vi "高级演示程序.vi"() -> ()   [LabVIEW 2012]
panel:
  out "存储中转":bool=TRUE
  in  "采样频率":i32=1000000
  in  "退出回放":bool
  out "zhongji":bool
  in  "退出系统":bool
  in  "触发时间":i32
  out "size":i32
  out "datafile":path[](array[path])
  in  "选项卡控件":enum32{"数据采集 ", "数字量采集", "数据回放"}(tab)
  out "实时波形显示":dbl[][](graph)
  out "当前状态":string
  in  "触发状态":bool
  in  "开始AD":bool
  in  "停止AD":bool
  in  "触发时间 2":i32 caption="mS"
  in  "定时":bool
  in  "触发按钮":bool
  in  "功能选项卡":enum32{"采集参数配置", "存储图形参数"}(tab)
  in  "M段":i32
  in  "N段":i32=40960
  in  "量程":T1(array[ring])
  in  "增益":enum16{"1倍", "2倍", "4倍", "8倍"}[](array[ring])
  in  "Y轴标尺调整":i8(knob) scale=0.0..10.0
  in  "文件名":string
  in  "存储":bool
  in  "触发方向":enum16{"下降沿触发", "上升沿触发", "上下边沿均触发"}(ring)
  in  "触发模式":enum16{"中间触发", "后触发", "预触发", "硬件延时触发"}(ring)
  in  "触发电平":i32
  in  "触发源":enum16{"软件触发", "DTR触发", "ATR触发", "Trig触发"}(ring)
  in  "时钟输出到总线":enum16{"不允许", "允许"}(ring)
  in  "时钟源":enum16{"内时钟", "外时钟"}(ring)
  in  "时钟输入输出源":T2(ring)
  in  "DO4":bool
  in  "DO5":bool
  in  "DO7":bool
  in  "DO6":bool
  in  "DO3":bool
  in  "DO2":bool
  in  "DO1":bool
  in  "DO0":bool
  out "DI7":bool
  out "DI6":bool
  out "DI5":bool
  out "DI4":bool
  out "DI3":bool
  out "DI2":bool
  out "DI1":bool
  out "DI0":bool
  in  "显示点数":u32(knob)=1000 min=1 max=10000 step=1000 scale=1.0..10000.0
  in  "刷新速度":u32(knob)=100 min=100 max=1000 step=100 scale=100.0..1000.0
  in  "开始":bool
  out "Waveform Graph 3":dbl[](graph)
  in  "导入":bool
  in  "循环速度（MS）":u32=300
  in  "量程-1":T3(ring)
  # "时钟源"
  # "触发方式"
  # "通道设置"
  # "数字量输出"
  # "数字量采集"
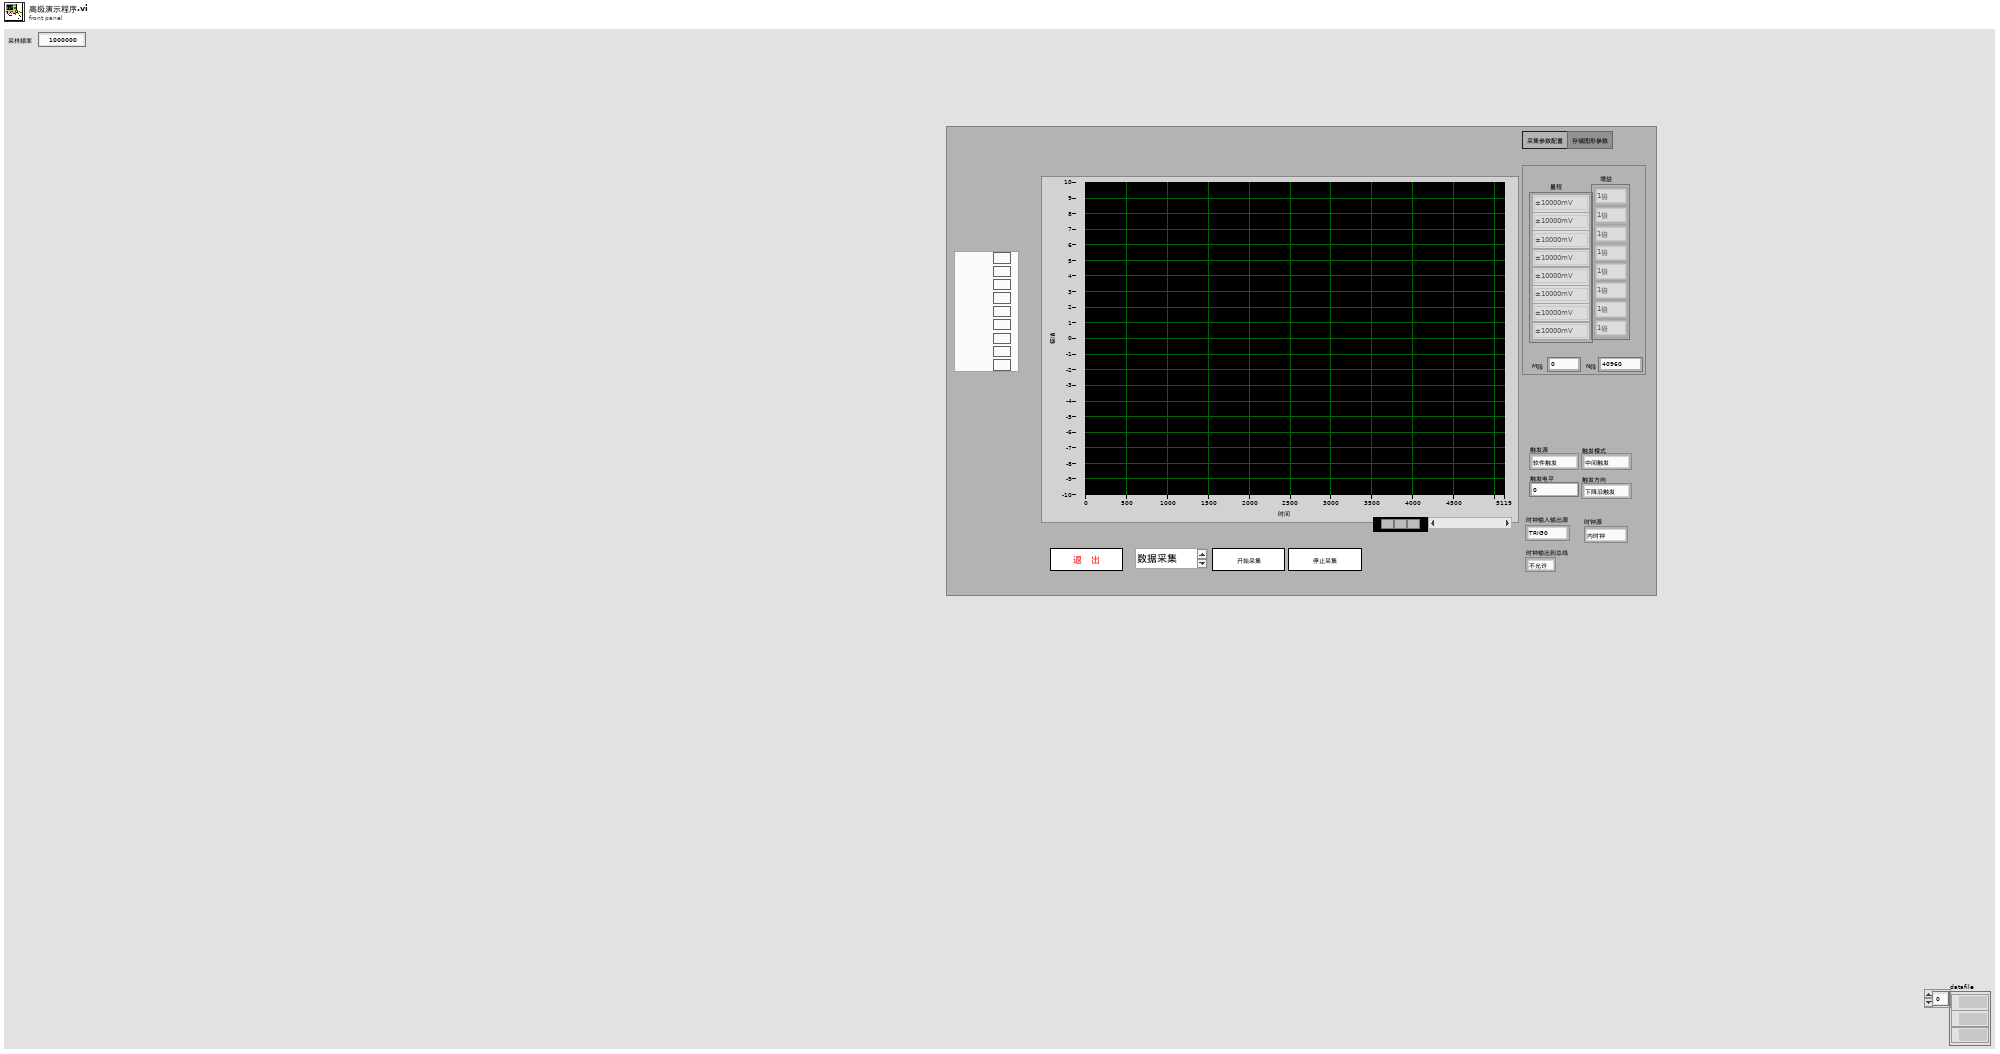
[diagram p1: front panel]
types:
  T1 = enum16{"±10000mV", "±5000mV", "±2500mV", "0-10000mV", "0-5000mV"}[]
  T2 = enum16{"TRIG0", "TRIG1", "TRIG2", "TRIG3", "TRIG4", "TRIG5", "TRIG6", "TRIG7"}
  T3 = enum16{"±10000mV", "±5000mV", "±2500mV", "0-10000mV", "0-5000mV"}
  T4 = enum8{"Enabled", "Disabled", "Disabled and Grayed Out"}
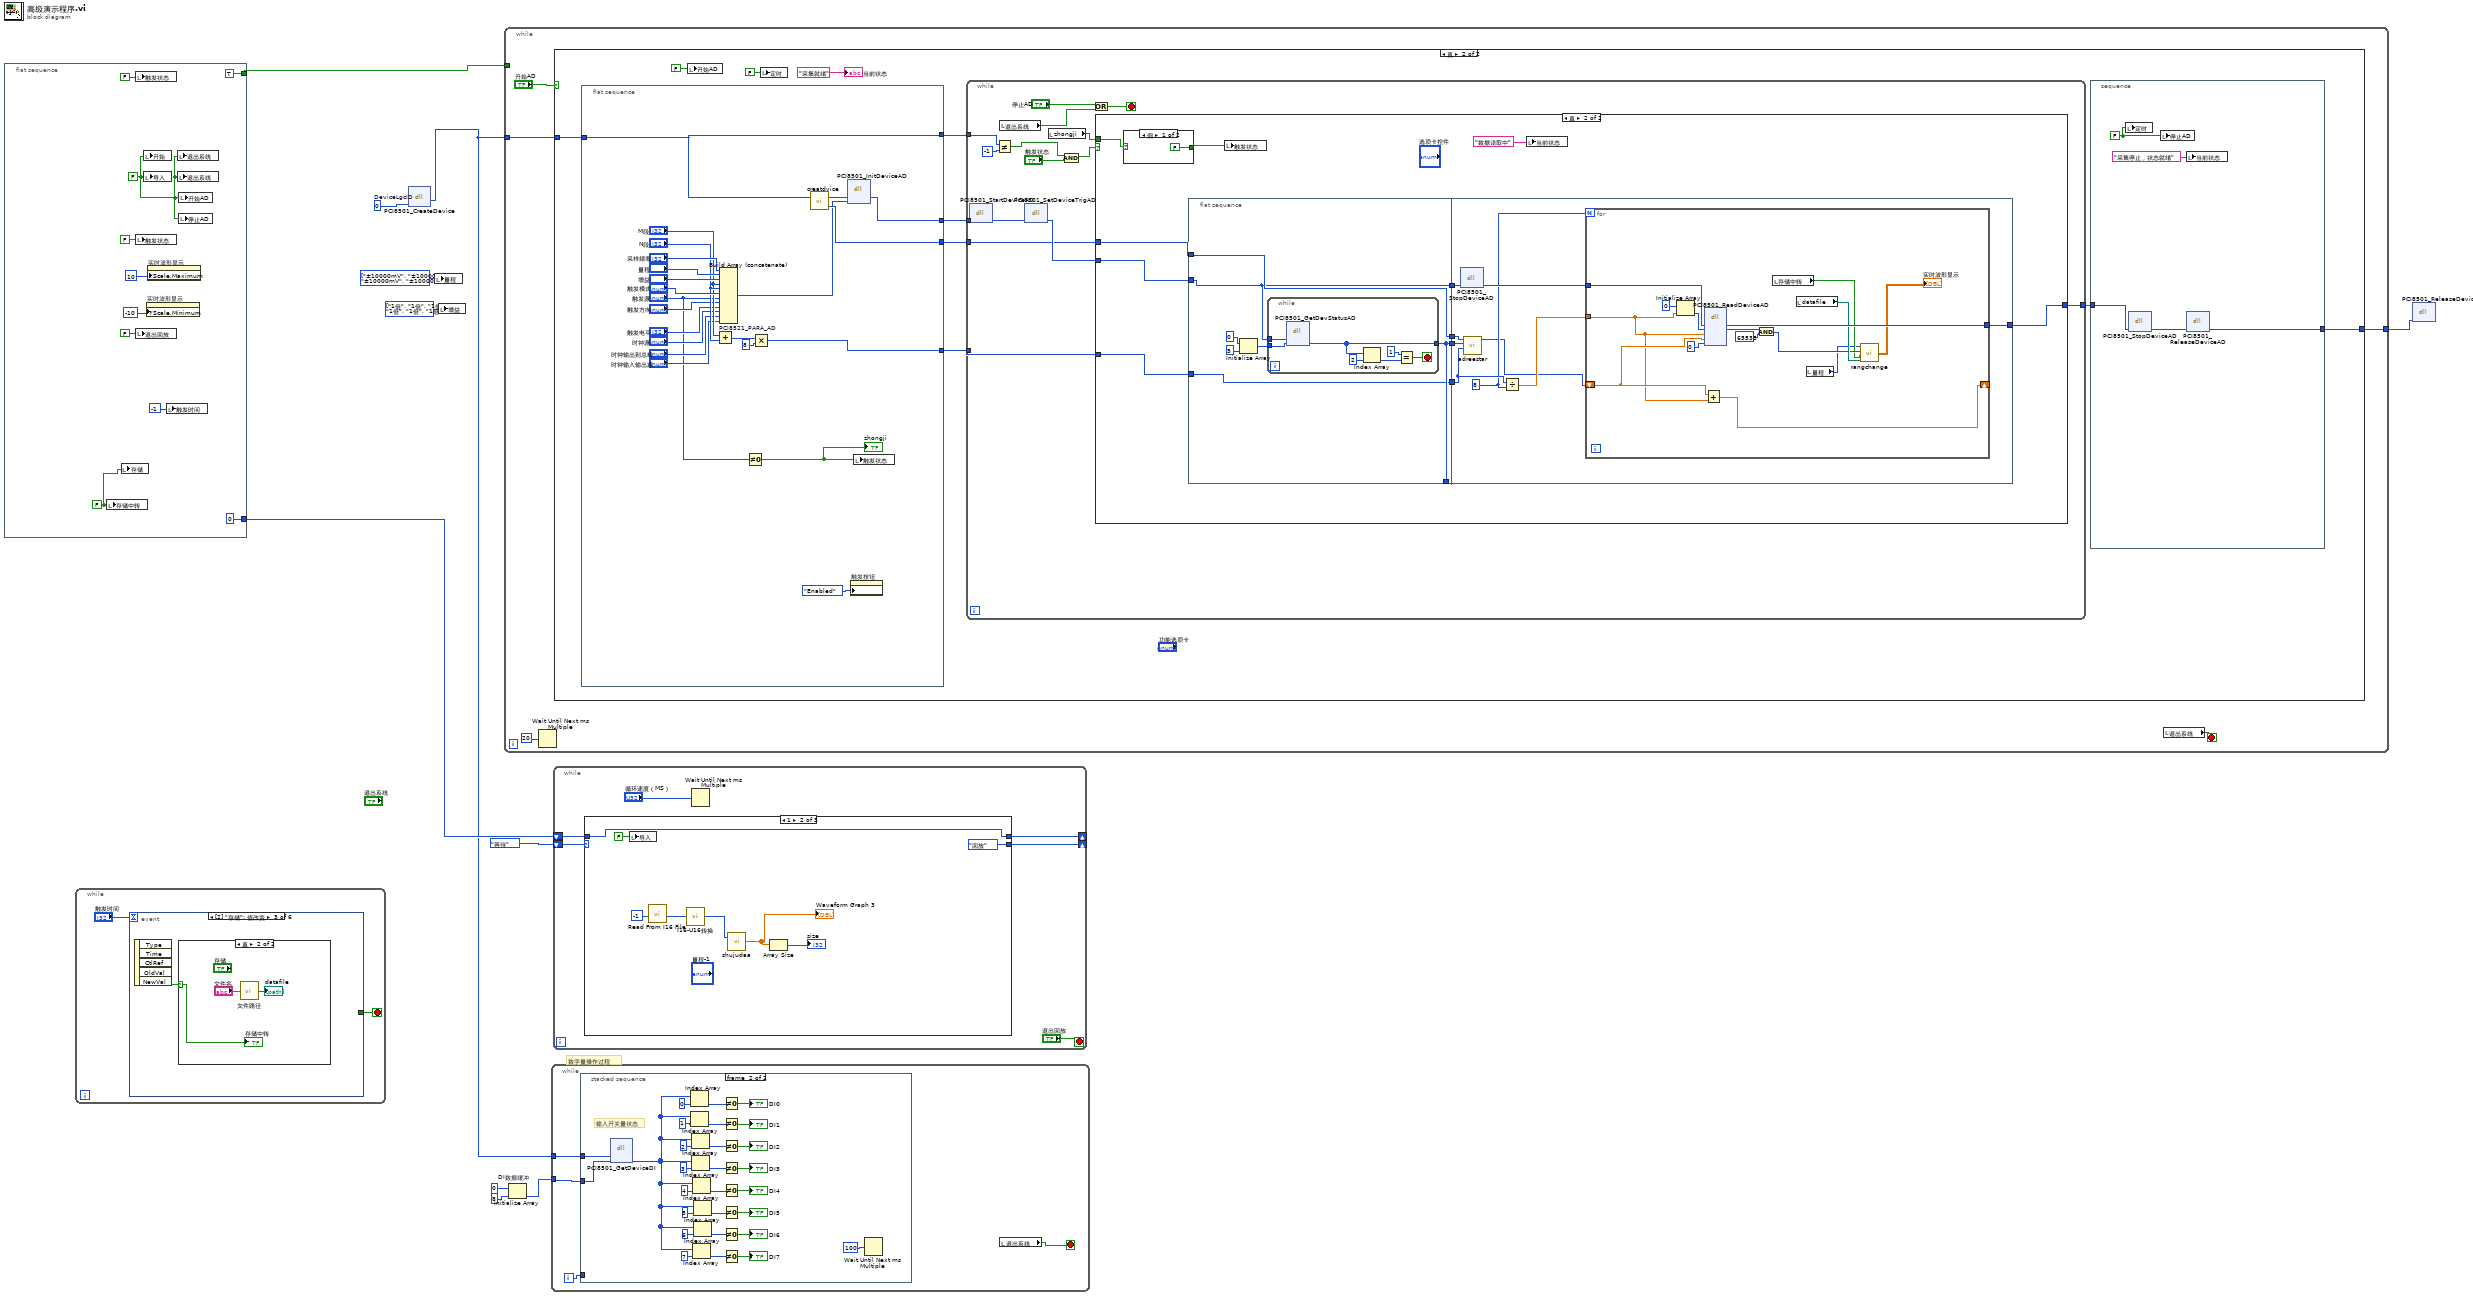
[diagram p0: block diagram]
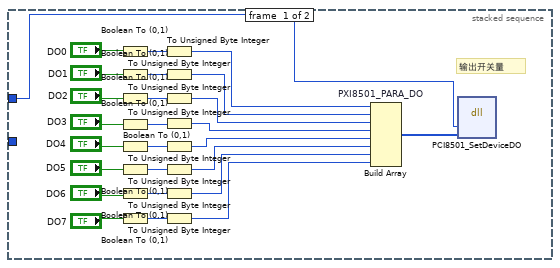
[diagram p2: hidden frame]
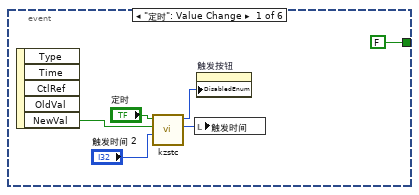
[diagram p3: hidden frame]
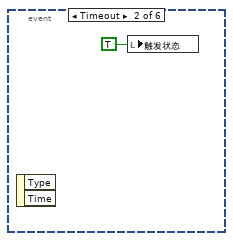
[diagram p4: hidden frame]
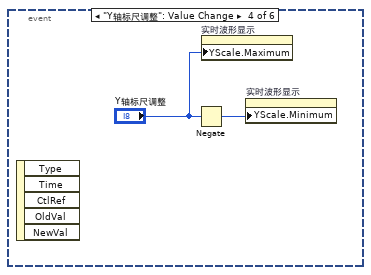
[diagram p6: hidden frame]
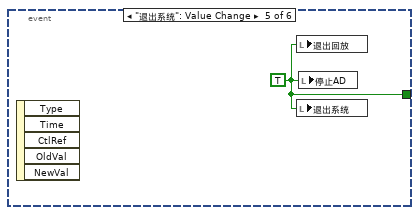
[diagram p7: hidden frame]
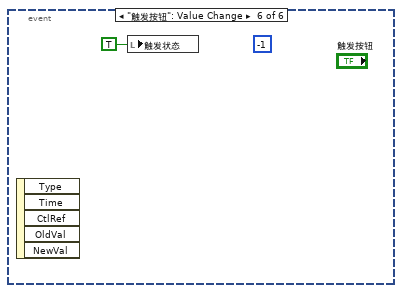
[diagram p8: hidden frame]
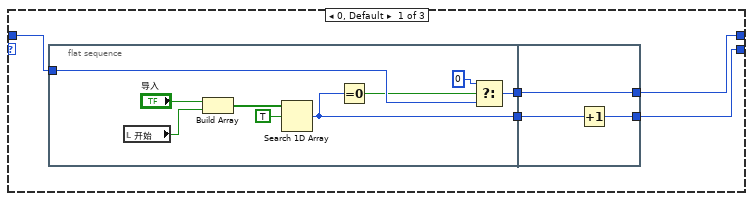
[diagram p9: hidden frame]
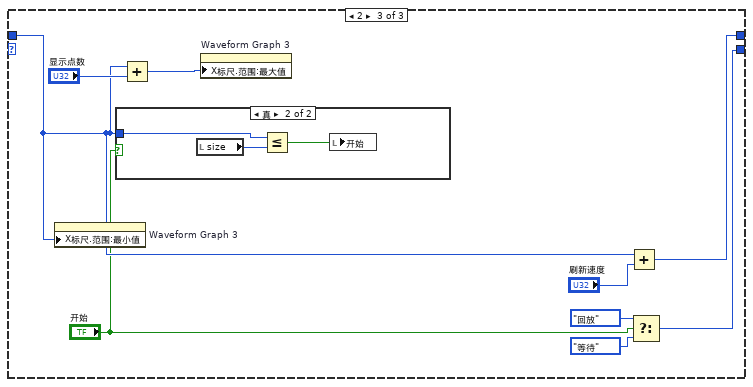
[diagram p10: hidden frame]
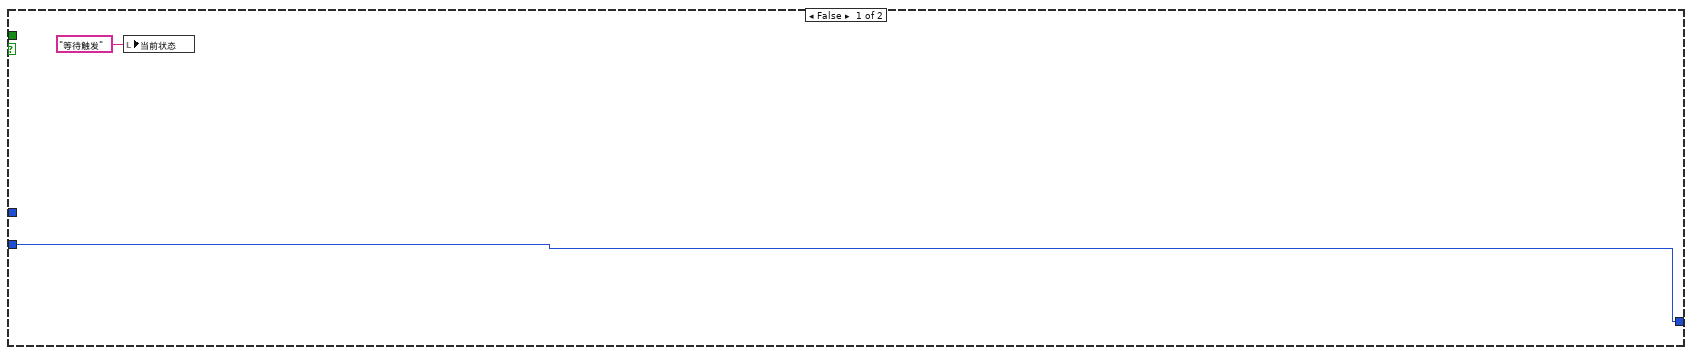
[diagram p13: hidden frame]
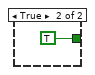
[diagram p14: hidden frame]
diagram:
  w1 = enum16{"1倍", "2倍", "4倍", "8倍"}[] [enum."1倍", enum."1倍", enum."1倍", enum."1倍", enum."1倍", enum."1倍", enum."1倍", enum."1倍"] items=["1倍", "2倍", "4倍", "8倍"] ("增益")
  w2 = T1 [enum."±10000mV", enum."±10000mV", enum."±10000mV", enum."±10000mV", enum."±10000mV", enum."±10000mV", enum."±10000mV", enum."±10000mV"] items=["±10000mV", "±5000mV", "±2500mV", "0-10000mV", "0-5000mV"] ("量程")
  w4 = 0  # DeviceLgcID
  # "数字量操作过程"
  n1 = flat-sequence {
    tunnel: [TRUE] -> w10
    tunnel: [0] -> w6
    frame #0 {
      w12 = FALSE ("存储中转")
      w18 = FALSE ("开始AD")
      n2 = local write "存储中转"(w12) -> ()
      n3 = local write "存储"(w12) -> ()
      n4 = local write "触发状态"(FALSE ("tirg")) -> ()
      n5 = local write "触发状态"(FALSE ("触发状态")) -> ()
      n6 = local write "退出回放"(FALSE ("退出回放")) -> ()
      n7 = local write "开始"(w18) -> ()
      n8 = local write "导入"(w18) -> ()
      n9 = property on="实时波形显示" class="WFGraph (严格)"("YScale.Minimum"=i8 -10 ("Y标尺.范围:最小值")) -> ()  [unwired: 2 in, 2 out]
      n10 = property on="实时波形显示" class="WFGraph (严格)"("YScale.Maximum"=u8 10 ("Y标尺.范围:最大值")) -> ()  [unwired: 2 in, 2 out]
      n11 = local write "触发时间"(-1 ("触发时间 2")) -> ()
      n12 = local write "退出系统"(w18) -> ()
      n13 = local write "退出系统"(w18) -> ()
      n14 = local write "开始AD"(w18) -> ()
      n15 = local write "停止AD"(w18) -> ()
    }
  }
  n16 = while {
    stop <- w23 stop-if-true
    n17 = event shown="[2] \"存储\": 值改变" {
      selector: _ -> [_ _ _ _ _ _]
      dyn-events: _ -> [_ _ _ _ _ _]
      timeout: "触发时间" -> [_ _ _ _ _ _]
      tunnel: [FALSE _ _ _ w37 _] -> w23
      event "定时": Value Change {
        n18 = event-data() -> ("NewVal"=w27:bool)  [unwired: 1 in, 4 out]
        n19 = call "kzstc.vi"("触发时间输入"="触发时间 2", "NewVal"=w27, "定时"="定时") -> ("触发时间输出"=w28:i32, "禁用"=w26:T4)  [unwired: 7 in]
        n20 = local write "触发时间"(w28) -> ()
        n21 = property on="触发按钮" class="Bool"("DisabledEnum"=w26) -> ()  [unwired: 2 in, 2 out]
      }
      event Timeout {
        n22 = event-data() -> ()  [unwired: 1 in, 2 out]
        n23 = local write "触发状态"(TRUE ("tirg")) -> ()
      }
      event "存储": Value Change {
        n24 = event-data() -> ("NewVal"=w31:bool)  [unwired: 1 in, 4 out]
        n25 = case shown="真" w31 {
          selector: w31 -> [_ w32]
          frame False {
          }
          frame True {
            n26 = call "文件路径.vi"("文件名"="文件名") -> ("数组"=→"datafile":path[])
            "存储中转" <- w32
          }
        }
      }
      event "Y轴标尺调整": Value Change {
        n27 = event-data() -> ()  [unwired: 1 in, 5 out]
        n28 = Negate(x="Y轴标尺调整") -> (-x=w36:i8)
        n29 = property on="实时波形显示" class="WFGraph (严格)"("YScale.Maximum"="Y轴标尺调整") -> ()  [unwired: 2 in, 2 out]
        n30 = property on="实时波形显示" class="WFGraph (严格)"("YScale.Minimum"=w36) -> ()  [unwired: 2 in, 2 out]
      }
      event "退出系统": Value Change {
        w37 = TRUE
        n31 = event-data() -> ()  [unwired: 1 in, 5 out]
        n32 = local write "退出回放"(w37) -> ()
        n33 = local write "退出系统"(w37) -> ()
        n34 = local write "停止AD"(w37) -> ()
      }
      event "触发按钮": Value Change {
        (unwired) -1 ("触发时间")
        n35 = event-data() -> ()  [unwired: 1 in, 5 out]
        n36 = local write "触发状态"(TRUE ("tirg")) -> ()
      }
    }
  }
  n37 = dll-call lib="PCI8501_32" fn="PCI8501_CreateDevice" label="CreateDevice"("DeviceLgcID"=w4) -> ("返回类型"=w3:i32)  [unwired: 4 in, 2 out]
  n38 = local write "量程"(w2) -> ()
  n39 = local write "增益"(w1) -> ()
  n40 = while {
    tunnel: w10 -> [_]
    tunnel: [w40] -> w5
    tunnel: w3 -> [w39]
    stop <- w43 stop-if-true
    n41 = Wait Until Next ms Multiple(millisecond multiple=u32 20 ("毫秒倍数")) -> ()  [unwired: 1 out]
    n42 = case shown="真" "开始AD" {
      tunnel: [_ w46] -> w40
      tunnel: w39 -> [_ w45]
      frame False {
      }
      frame True {
        n43 = flat-sequence {
          tunnel: [w55] -> w53
          tunnel: [w72] -> w49
          tunnel: [w71] -> w48
          tunnel: w45 -> [w70]
          tunnel: [w70] -> w44
          frame #0 {
            n44 = Add(x="M段", y="N段") -> (x+y=w69:i32)
            n45 = Build Array (concatenate) "PCI8521_PARA_AD"("采样频率", "量程", "增益", "M段", "N段", "触发模式", "触发源", "触发方向", "触发电平", "时钟源", "时钟输出到总线", "时钟输入输出源") -> (w56:i32[])
            n46 = Not Equal To 0?(x="触发源") -> (x != 0?=w75:bool)
            "zhongji" <- w75
            n47 = Multiply(x=w69, y=8 ("element")) -> (x*y=w55:i32)
            n48 = call "creatdvice.vi"("数值"=w70) -> ("ddrlength"=w71:i32, "hDevice"=w73:i32)  [unwired: 1 in]
            n49 = dll-call lib="PCI8501_32" fn="PCI8501_InitDeviceAD" label="InitDeviceAD"("hDevice"=w73, "pADPara"=w56) -> ("hDevice"=w72:i32)  [unwired: 5 in, 2 out]
            n50 = property on="触发按钮" class="Bool"("DisabledEnum"=T4."Enabled" ("禁用")) -> ()  [unwired: 2 in, 2 out]
            n51 = local write "触发状态"(w75) -> ()
          }
        }
        n52 = local write "开始AD"(FALSE ("开始AD")) -> ()
        n53 = local write "定时"(FALSE ("定时")) -> ()
        n54 = while {
          tunnel: w53 -> [w78]
          tunnel: w49 -> [w81]
          tunnel: w48 -> [w79]
          tunnel: [w77] -> w47
          tunnel: w44 -> [w76]
          stop <- w87 stop-if-true
          n55 = dll-call lib="PCI8501_32" fn="PCI8501_StartDeviceAD" label="StartDeviceAD"("hDevice"=w81) -> ("hDevice"=w82:i32)  [unwired: 4 in, 2 out]
          n56 = Not Equal?(x=w76, y=-1) -> (x != y?=w86:bool)
          n57 = local read "退出系统"() -> (w88:bool)
          n58 = dll-call lib="PCI8501_32" fn="PCI8501_SetDeviceTrigAD" label="SetDeviceTrigAD"("hDevice"=w82) -> ("hDevice"=w80:i32)  [unwired: 4 in, 2 out]
          n59 = local read "zhongji"() -> (w83:bool)
          n60 = Compound Arithmetic op=AND(w86, "触发状态") -> (w85:bool)
          n61 = Or(x="停止AD", y=w88) -> (x .or. y?=w87:bool)
          n62 = case shown="真" w85 {
            tunnel: w83 -> [_ w102]
            tunnel: w80 -> [w91 w96]
            tunnel: w79 -> [_ w95]
            tunnel: w78 -> [_ w94]
            tunnel: [w91 w93] -> w77
            frame False {
              n63 = local write "当前状态"("等待触发" ("当前状态")) -> ()
            }
            frame True {
              n64 = case shown="假" w102 {
                tunnel: [FALSE ("触发状态") TRUE ("触发状态")] -> w103
                frame False {
                }
                frame True {
                }
              }
              n65 = flat-sequence {
                tunnel: [w104] -> w100
                tunnel: [w107] -> _
                tunnel: w94 -> [w106]
                tunnel: [w106] -> w99
                tunnel: w95 -> [w105]
                tunnel: [w105] -> w98
                tunnel: [w107] -> w97
                tunnel: w96 -> [w104]
                tunnel: w100 -> [w126]
                tunnel: [w124] -> w93
                tunnel: w99 -> [w121]
                tunnel: w98 -> [w122]
                tunnel: w97 -> [w123]
                frame #0 {
                  n66 = Initialize Array(0, 5) -> (w110:i32[])
                  n67 = while {
                    tunnel: w104 -> [w117]
                    tunnel: w110 -> [w116]
                    tunnel: [w111] -> w107
                    stop <- w112 stop-if-true
                    n68 = dll-call lib="PCI8501_32" fn="PCI8501_GetDevStatusAD" label="GetDevStatusAD"("hDevice"=w117, "ADStatus"=w116) -> ("ADStatus"=w111:i32[])  [unwired: 5 in, 2 out]
                    n69 = Index Array(array=w111, index=2) -> (element=w114:i32)
                    n70 = Equal?(x=1, y=w114) -> (x = y?=w112:bool)
                  }
                }
                frame #1 {
                  w120 = 8 ("y")
                  n71 = dll-call lib="PCI8501_32" fn="PCI8501_StopDeviceAD" label="StopDeviceAD"("hDevice"=w126) -> ("hDevice"=w125:i32)  [unwired: 4 in, 2 out]
                  n72 = call "adreestar.vi"("M+N*8"=w121, "ADStatus"=w123, "ddrlength"=w122) -> ("adree"=w118:i32)  [unwired: 8 in]
                  n73 = Divide(x=w121, y=w120) -> (x/y=w119:dbl)
                  n74 = for {
                    N: w120 -> [_]
                    tunnel: w125 -> [w137]
                    tunnel: [w135] -> w124
                    shift-right: [w132] -> _
                    shift-left: w118 -> [w134]
                    tunnel: w119 -> [w133]
                    n75 = Initialize Array(0 ("y"), w133) -> (w139:i32[])
                    n76 = dll-call lib="PCI8501_32" fn="PCI8501_ReadDeviceAD" label="ReadDeviceAD"("hDevice"=w137, "ADBuffer"=w139, "AD_DATA_LEN"=w133, "ulStartAddr"=w134, "nRetSizeWords"=0 ("y")) -> ("hDevice"=w135:i32, "ADBuffer"=w136:u16[])  [unwired: 7 in, 2 out]
                    n77 = Add(x=w134, y=w133) -> (x+y=w132:dbl)
                    n78 = And(x=w136, y=65535) -> (x .and. y?=w129:i32[])
                    n79 = local read "存储中转"() -> (w128:bool)
                    n80 = local read "datafile"() -> (w131:path[])
                    n81 = local read "量程"() -> (w127:T1)
                    n82 = call "rangchange.vi"("datafile"=w131, "savaen"=w128, "IN"=w129, "添加的数组 2"=w127) -> ("添加的数组"=→"实时波形显示":dbl[][])  [unwired: 2 in]
                  }
                }
              }
              n83 = local write "触发状态"(w103) -> ()
              n84 = local write "当前状态"("数据读取中" ("当前状态")) -> ()
            }
          }
        }
        n85 = stacked-sequence {
          tunnel: w47 -> [w145]
          tunnel: [w144] -> w46
          frame #0 {
            w148 = FALSE ("停止AD")
            n86 = local write "定时"(w148) -> ()
            n87 = dll-call lib="PCI8501_32" fn="PCI8501_StopDeviceAD" label="StopDeviceAD"("hDevice"=w145) -> ("hDevice"=w146:i32)  [unwired: 4 in, 2 out]
            n88 = local write "停止AD"(w148) -> ()
            n89 = local write "当前状态"("采集停止，状态就绪" ("当前状态")) -> ()
            n90 = dll-call lib="PCI8501_32" fn="PCI8501_ReleaseDeviceAD" label="ReleaseDeviceAD"("hDevice"=w146) -> ("hDevice"=w144:i32)  [unwired: 4 in, 2 out]
          }
        }
        "当前状态" <- "采集就绪" ("当前状态")
      }
    }
    n91 = local read "退出系统"() -> (w43:bool)
  }
  n92 = Initialize Array "DI数据缓冲"(u8 0 ("元素初值"), 8) -> (w7:u8[])
  n93 = while {
    tunnel: w7 -> [w152]
    tunnel: w3 -> [w149]
    i -> [w151]
    stop <- w150 stop-if-true
    n94 = stacked-sequence {
      tunnel: w152 -> [_ w182]
      tunnel: w151 -> [_ _]
      tunnel: w149 -> [w153 w179]
      frame #0 {
        # "输出开关量"
        n95 = Boolean To (0,1)(Boolean="DO0") -> (0, 1=w170:i16)
        n96 = Boolean To (0,1)(Boolean="DO1") -> (0, 1=w178:i16)
        n97 = Boolean To (0,1)(Boolean="DO2") -> (0, 1=w175:i16)
        n98 = Boolean To (0,1)(Boolean="DO3") -> (0, 1=w169:i16)
        n99 = Boolean To (0,1)(Boolean="DO4") -> (0, 1=w174:i16)
        n100 = Boolean To (0,1)(Boolean="DO5") -> (0, 1=w173:i16)
        n101 = Boolean To (0,1)(Boolean="DO6") -> (0, 1=w172:i16)
        n102 = Boolean To (0,1)(Boolean="DO7") -> (0, 1=w171:i16)
        n103 = To Unsigned Byte Integer(number=w170) -> (unsigned 8bit integer=w168:u8)
        n104 = To Unsigned Byte Integer(number=w178) -> (unsigned 8bit integer=w167:u8)
        n105 = To Unsigned Byte Integer(number=w175) -> (unsigned 8bit integer=w166:u8)
        n106 = To Unsigned Byte Integer(number=w169) -> (unsigned 8bit integer=w165:u8)
        n107 = To Unsigned Byte Integer(number=w174) -> (unsigned 8bit integer=w164:u8)
        n108 = To Unsigned Byte Integer(number=w173) -> (unsigned 8bit integer=w163:u8)
        n109 = To Unsigned Byte Integer(number=w172) -> (unsigned 8bit integer=w162:u8)
        n110 = To Unsigned Byte Integer(number=w171) -> (unsigned 8bit integer=w161:u8)
        n111 = Build Array "PXI8501_PARA_DO"(w168, w167, w166, w165, w164, w163, w162, w161) -> (w154:u8[])
        n112 = dll-call lib="PCI8501_32" fn="PCI8501_SetDeviceDO" label="SetDeviceDO"("hDevice"=w153, "bDOSts"=w154) -> ()  [unwired: 6 in, 2 out]
      }
      frame #1 {
        # "输入开关量状态"
        n113 = dll-call lib="PCI8501_32" fn="PCI8501_GetDeviceDI" label="GetDeviceDI"("hDevice"=w179, "bDISts"=w182) -> ("bDISts"=w181:u8[])  [unwired: 5 in, 2 out]
        n114 = Index Array(array=w181, index=0) -> (element=w197:u8)
        n115 = Index Array(array=w181, index=1) -> (element=w198:u8)
        n116 = Index Array(array=w181, index=2) -> (element=w196:u8)
        n117 = Index Array(array=w181, index=3) -> (element=w195:u8)
        n118 = Index Array(array=w181, index=4) -> (element=w194:u8)
        n119 = Index Array(array=w181, index=7) -> (element=w191:u8)
        n120 = Index Array(array=w181, index=5) -> (element=w193:u8)
        n121 = Index Array(array=w181, index=6) -> (element=w192:u8)
        n122 = Not Equal To 0?(x=w197) -> (x != 0?=→"DI0":bool)
        n123 = Not Equal To 0?(x=w198) -> (x != 0?=→"DI1":bool)
        n124 = Not Equal To 0?(x=w196) -> (x != 0?=→"DI2":bool)
        n125 = Not Equal To 0?(x=w195) -> (x != 0?=→"DI3":bool)
        n126 = Not Equal To 0?(x=w194) -> (x != 0?=→"DI4":bool)
        n127 = Not Equal To 0?(x=w193) -> (x != 0?=→"DI5":bool)
        n128 = Not Equal To 0?(x=w192) -> (x != 0?=→"DI6":bool)
        n129 = Not Equal To 0?(x=w191) -> (x != 0?=→"DI7":bool)
        n130 = Wait Until Next ms Multiple(millisecond multiple=u32 100) -> ()  [unwired: 1 out]
      }
    }
    n131 = local read "退出系统"() -> (w150:bool)
  }
  n132 = while {
    shift-right: [w210] -> _
    shift-left: w6 -> [w208]
    shift-right: [w211] -> _
    shift-left: enum16{"等待", "导入", "回放", "停止"}."等待" -> [w212]
    stop <- "退出回放" stop-if-true
    n133 = case shown="1" w212 {
      tunnel: [w216 enum16{"等待", "导入", "回放", "停止"}."回放" w244] -> w211
      tunnel: w208 -> [w215 w236 w241]
      tunnel: [w213 w236 w242] -> w210
      frame 0, Default {
        n134 = flat-sequence {
          tunnel: [w222] -> w217
          tunnel: w215 -> [w221]
          tunnel: [w220] -> w214
          tunnel: w217 -> [w229]
          tunnel: [w228] -> w216
          tunnel: [w227] -> w213
          tunnel: w214 -> [w227]
          frame #0 {
            n135 = local read "开始"() -> (w218:bool)
            n136 = Build Array("导入", w218) -> (w225:bool[])
            n137 = Search 1D Array(1D array=w225, element=TRUE) -> (index of element=w222:i32)  [unwired: 1 in]
            n138 = Equal To 0?(x=w222) -> (x = 0?=w219:bool)
            n139 = Select(t=0, s=w219, f=w221) -> (s? t:f=w220:u32)
          }
          frame #1 {
            n140 = Increment(x=w229) -> (x+1=w228:i32)
          }
        }
      }
      frame 1 {
        n141 = local write "导入"(FALSE ("导入")) -> ()
        n142 = call <vilib>:"Read From I16 File.vi"("2D number of columns/1D count (all as 1D:-1)"=-1) -> ("1D array"=w230:i16[])  [unwired: 6 in, 4 out]
        n143 = call "I16-U16转换.vi"("输入"=w230) -> ("输出"=w232:i32[])
        n144 = call "shujudaa.vi"("inputdata"=w232) -> ("outdata"=w231:dbl[])  [unwired: 1 in]
        "Waveform Graph 3" <- w231
        n145 = Array Size(array=w231) -> (size(s)=→"size":i32)
      }
      frame 2 {
        n146 = property on="Waveform Graph 3" class="WFGraph (严格)"("X标尺.范围:最小值"=w241) -> ()  [unwired: 2 in, 2 out]
        n147 = case shown="真" "开始" {
          tunnel: w241 -> [_ w249]
          frame False {
          }
          frame True {
            n148 = local read "size"() -> (w247:i32)
            n149 = Less Or Equal?(x=w249, y=w247) -> (x <= y?=w248:bool)
            n150 = local write "开始"(w248) -> ()
          }
        }
        n151 = Add(x=w241, y="显示点数") -> (x+y=w243:u32)
        n152 = property on="Waveform Graph 3" class="WFGraph (严格)"("X标尺.范围:最大值"=w243) -> ()  [unwired: 2 in, 2 out]
        n153 = Add(x=w241, y="刷新速度") -> (x+y=w242:u32)
        n154 = Select(t=enum16{"等待", "导入", "回放", "停止"}."回放", s="开始", f=enum16{"等待", "导入", "回放", "停止"}."等待") -> (s? t:f=w244:enum16{"等待", "导入", "回放", "停止"})
      }
    }
    n155 = Wait Until Next ms Multiple(millisecond multiple="循环速度（MS）") -> ()  [unwired: 1 out]
  }
  n156 = dll-call lib="PCI8501_32" fn="PCI8501_ReleaseDevice" label="ReleaseDevice"("hDevice"=w5) -> ()  [unwired: 5 in, 2 out]
